vi "Turbo.vi"(2 "Turbo":bool, 3 "error in (no error)":errorcluster, 4 "Right axis value":dbl, 5 "Left axis value":dbl) -> (0 "error out":errorcluster, 1 "Motor Values":dbl[](array[numeric]))   [LabVIEW 2012]
uses:
  <vilib>/Rock Robotics/WPI/RobotDrive/WPI_RobotDriveGetSetRefNum.vi
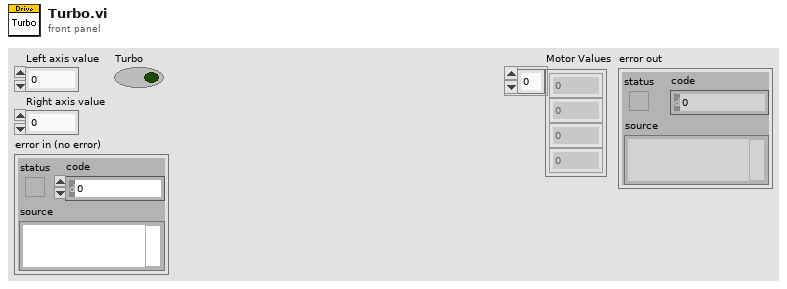
[diagram p1: front panel]
types:
  T1 = typedef "WPI_RobotDriveDevRef.ctl" = cluster{"DevStatus":errorcluster, "Motors[]":T2[], "Square Inputs":bool, "Max Output":dbl, "Isochronous":bool}
  T2 = typedef "WPI_MotorControlDeviceRef.ctl" = cluster{"DeviceStatus":errorcluster, "Type":enum16{"PWM", "CAN"}, "PWM":cluster{"Digital Module":T3, "PWM Channel":T4, "DeadBand":T5}, "CAN":cluster{"Device Number":u8, "Control Mode":T6, "Semaphore":T7, "Max Vout":dbl}, "Invert":bool, "TransformRef":T8, "InvTransformRef":T8}
  T3 = typedef "FPGA_TypedefDigitalModule.ctl" = enum16{"Digital Module 1", "Digital Module 2"}
  T4 = typedef "FPGA_DIOPWMChannel.ctl" = enum8{"PWM 1", "PWM 2", "PWM 3", "PWM 4", "PWM 5", "PWM 6", "PWM 7", "PWM 8", "PWM 9", "PWM 10", "Invalid"}
  T5 = typedef "WPI_PWMDeadband.ctl" = cluster{"Name":string, "maxPositivePwm":i32, "minPositivePwm":i32, "centerPwm":i32, "maxNegativePwm":i32, "minNegativePwm":i32, "angularRange":u16}
  T6 = typedef "WPI_CANJaguar_ControlMode.ctl" = enum8{"Percent VBus", "Current", "Speed", "Position", "Voltage"}
  T7 = typedef "Semaphore RefNum" = refnum<k1>
  T8 = typedef "WPI_PWMTransform_ConPane.ctl" = refnum<vi>
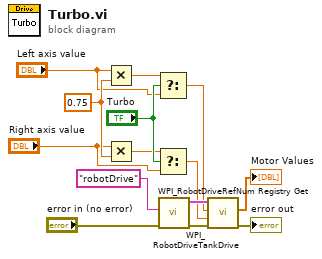
[diagram p0: block diagram]
diagram:
  w5 = 0.75 ("y")
  n1 = Multiply(x="Left axis value", y=w5) -> (x*y=w2:dbl)
  n2 = Multiply(x="Right axis value", y=w5) -> (x*y=w4:dbl)
  n3 = Select(t=w2, s="Turbo", f="Left axis value") -> (s? t:f=w12:dbl)
  n4 = Select(t=w4, s="Turbo", f="Right axis value") -> (s? t:f=w10:dbl)
  n5 = call <vilib>:"WPI_RobotDriveRefNum Registry Get.vi"("error in (no error)"="error in (no error)", "refnum name"="robotDrive") -> ("error out"=w8:errorcluster, "RobotDriveDevRef"=w13:T1)  [unwired: 8 out]
  n6 = call <vilib>:"WPI_RobotDriveTankDrive.vi"("error in (no error)"=w8, "Right axis value"=w10, "Left axis value"=w12, "RobotDriveDevRef"=w13) -> ("error out"=→"error out":errorcluster, "Motor Values"=→"Motor Values":dbl[])  [unwired: 5 in, 1 out]
